vi "backup.vi"() -> ()   [LabVIEW 2018]
uses:
  spi_instructions.ctl
  packet_type_t.ctl
  packet_t.ctl
  grabber_register_addr.ctl
  Seven_seg_disp.xctl
panel:
  in  "Colors [4]":cluster{u32, u32}[](array[cluster]) {"?" format="%x"}
  out "*(type *) &x 3":T1 {"instruction" items=["default"=0, "write"=173, "read"=237, "clear"=205]; "data" format="%x"; "address" format="%x"}
  out "Seven_seg_disp 16":u8(xcontrol)
  out "Seven_seg_disp 15":u8(xcontrol)
  out "Seven_seg_disp 14":u8(xcontrol)
  out "Seven_seg_disp 13":u8(xcontrol)
  out "Seven_seg_disp 12":u8(xcontrol)
  out "Seven_seg_disp 11":u8(xcontrol)
  out "Seven_seg_disp 10":u8(xcontrol)
  out "Seven_seg_disp 9":u8(xcontrol)
  out "LED15-8 2":bool[](array[boolean])
  out "LED7-0 2":bool[](array[boolean])
  out "unsigned byte array 2":u8[](array[numeric]) format="%x"
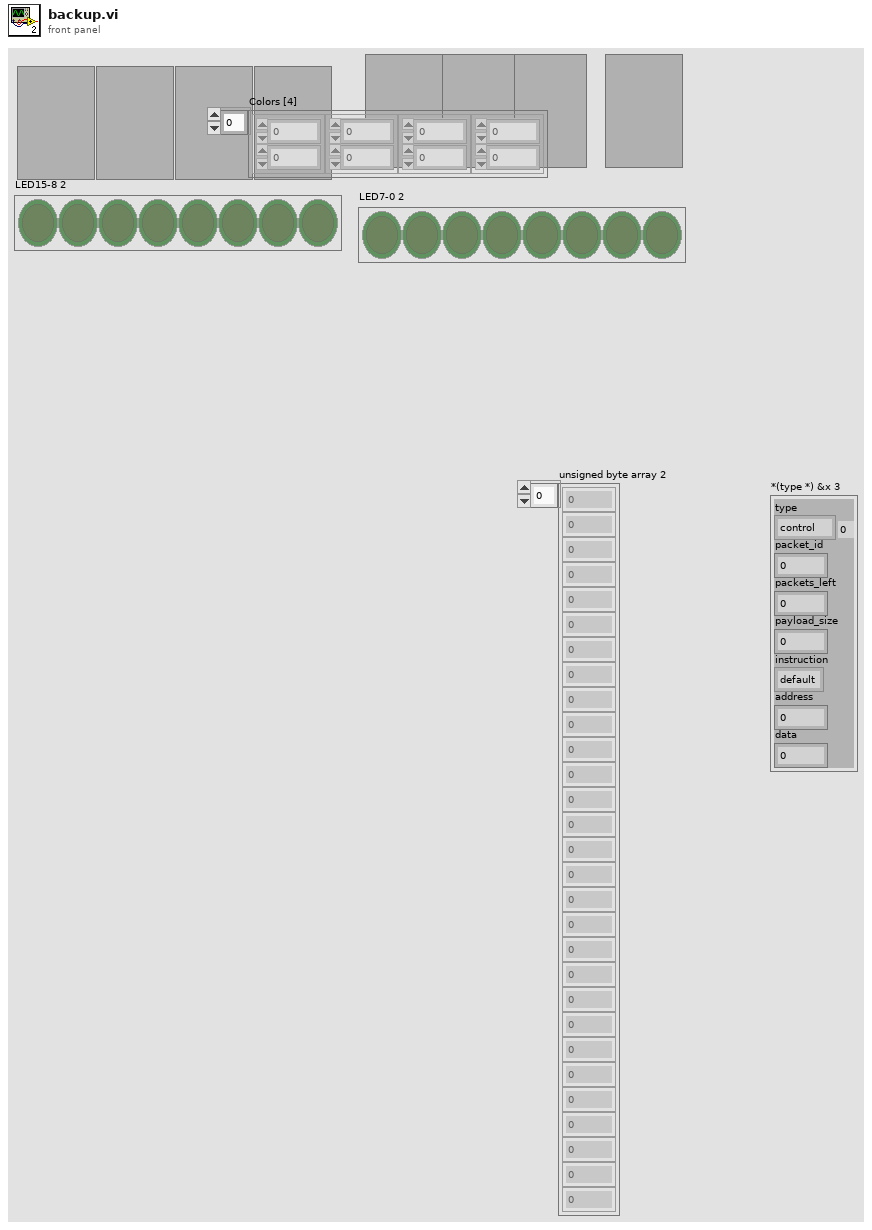
[diagram p1: front panel]
types:
  T1 = typedef "packet_t.ctl" = cluster{"type":T2, "packet_id":u16, "packets_left":u16, "payload_size":u16, "instruction":T3, "address":u8, "data":u8}
  T2 = typedef "packet_type_t.ctl" = enum8{"control", "spi", "audio", "hdmi"}
  T3 = typedef "spi_instructions.ctl" = u8
  T4 = typedef "grabber_register_addr.ctl" = enum8{"rgb_data", "led_data_low", "led_data_high", "digit_0_data", "digit_1_data", "digit_2_data", "digit_3_data", "digit_4_data", "digit_5_data", "digit_6_data", "digit_7_data"}
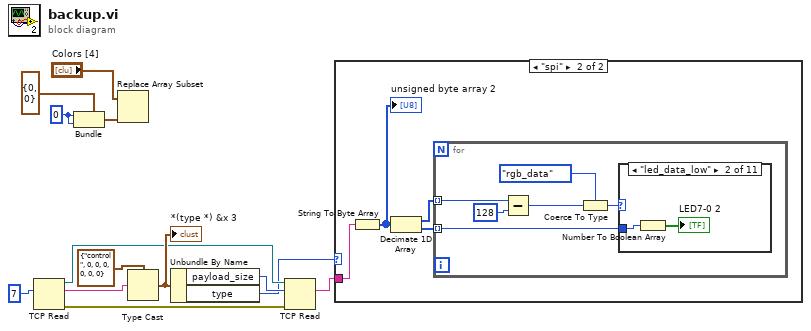
[diagram p0: block diagram]
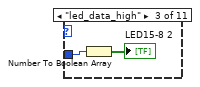
[diagram p4: hidden frame]
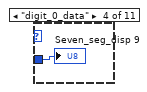
[diagram p5: hidden frame]
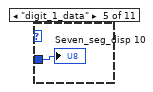
[diagram p6: hidden frame]
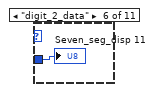
[diagram p7: hidden frame]
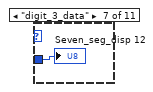
[diagram p8: hidden frame]
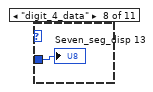
[diagram p9: hidden frame]
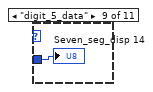
[diagram p10: hidden frame]
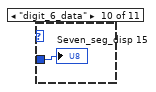
[diagram p11: hidden frame]
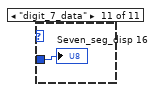
[diagram p12: hidden frame]
diagram:
  w1 = u32 0
  n1 = TCP Read(bytes to read=7) -> (connection ID=w5:refnum<k5>, connection ID out=w11:refnum<k5>, data out=w15:string, error out=w8:errorcluster)  [unwired: 3 in]
  n2 = Bundle(cluster=cluster{u32, u32} {0, 0}, w1, w1) -> (w4:cluster{u32, u32})
  n3 = Replace Array Subset(array="Colors [4]", new element=w4) -> ()  [unwired: 1 in, 1 out]
  n4 = Type Cast(type=T1 {"type"=enum."control", "packet_id"=0, "packets_left"=0, "payload_size"=0, "instruction"=0, "address"=0, "data"=0} ("element 2"), x=w15) -> (*(type *) &x=w13:T1)
  "*(type *) &x 3" <- w13
  n5 = Unbundle By Name(w13) -> ("payload_size"=w12:u16, "type"=w10:T2)
  n6 = TCP Read(connection ID=w11, bytes to read=w12, error in (no error)=w8) -> (connection ID out=w7:refnum<k5>, data out=w9:string, error out=w6:errorcluster)  [unwired: 2 in]
  n7 = case shown="\"spi\"" w10 {
    tunnel: w9 -> [_ w20]
    frame "control", Default {
    }
    frame "spi" {
      n8 = String To Byte Array(string=w20) -> (unsigned byte array=w19:u8[])
      "unsigned byte array 2" <- w19
      n9 = Decimate 1D Array(w19) -> (w18:u8[], w17:u8[])
      n10 = for {
        tunnel: w18 -> [w22] mode=indexing
        tunnel: w17 -> [w26] mode=indexing
        n11 = Subtract(x=w22, y=u8 128 ("x")) -> (x-y=w23:u8)
        n12 = Coerce To Type(0:w23, 1:grabber_register_addr."rgb_data" ("Enum")) -> (2:w24:T4)
        n13 = case shown="\"led_data_low\"" w24 {
          tunnel: w26 -> [_ w28 w30 w31 w32 w33 w34 w35 w36 w37 w38]
          frame "rgb_data", Default {
          }
          frame "led_data_low" {
            n14 = Number To Boolean Array(number=w28) -> (Boolean array=→"LED7-0 2":bool[])
          }
          frame "led_data_high" {
            n15 = Number To Boolean Array(number=w30) -> (Boolean array=→"LED15-8 2":bool[])
          }
          frame "digit_0_data" {
            "Seven_seg_disp 9" <- w31
          }
          frame "digit_1_data" {
            "Seven_seg_disp 10" <- w32
          }
          frame "digit_2_data" {
            "Seven_seg_disp 11" <- w33
          }
          frame "digit_3_data" {
            "Seven_seg_disp 12" <- w34
          }
          frame "digit_4_data" {
            "Seven_seg_disp 13" <- w35
          }
          frame "digit_5_data" {
            "Seven_seg_disp 14" <- w36
          }
          frame "digit_6_data" {
            "Seven_seg_disp 15" <- w37
          }
          frame "digit_7_data" {
            "Seven_seg_disp 16" <- w38
          }
        }
      }
    }
  }
